vi "Analysis.Folders.Initialize.vi"(11 "Parameters in":T1) -> (3 "Parameters out":T1)   [LabVIEW 2015, in "NIAnalysis.lvlib"]
uses:
  NIAnalysis.lvlib
  Types/AnalysisGUI.Parameters.ctl
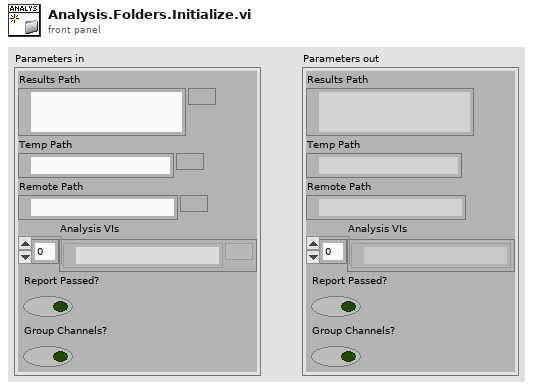
[diagram p1: front panel]
types:
  T1 = typedef "NIAnalysis.lvlib/AnalysisGUI.Parameters.ctl" = cluster{"Results Path":path, "Temp Path":path, "Remote Path":path, "Analysis VIs":path[], "Report Passed?":bool, "Group Channels?":bool}
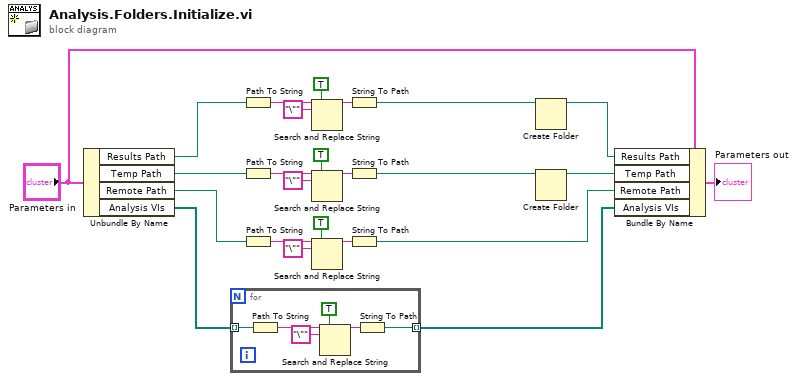
[diagram p0: block diagram]
diagram:
  n1 = Unbundle By Name("Parameters in") -> ("Results Path"=w2:path, "Temp Path"=w4:path, "Remote Path"=w6:path, "Analysis VIs"=w19:path[])
  n2 = for {
    tunnel: w19 -> [w26] mode=indexing
    tunnel: [w25] -> w23 mode=indexing
    n3 = Path To String(path=w26) -> (string=w29:string)
    n4 = Search and Replace String(replace all?=TRUE ("replace all? (F)"), input string=w29, search string="\"") -> (result string=w30:string)  [unwired: 5 in, 3 out]
    n5 = String To Path(string=w30) -> (path=w25:path)
  }
  n6 = Path To String(path=w2) -> (string=w17:string)
  n7 = Path To String(path=w4) -> (string=w13:string)
  n8 = Path To String(path=w6) -> (string=w9:string)
  n9 = Search and Replace String(replace all?=TRUE ("replace all? (F)"), input string=w17, search string="\"") -> (result string=w18:string)  [unwired: 5 in, 3 out]
  n10 = Search and Replace String(replace all?=TRUE ("replace all? (F)"), input string=w13, search string="\"") -> (result string=w14:string)  [unwired: 5 in, 3 out]
  n11 = Search and Replace String(replace all?=TRUE ("replace all? (F)"), input string=w9, search string="\"") -> (result string=w10:string)  [unwired: 5 in, 3 out]
  n12 = String To Path(string=w18) -> (path=w1:path)
  n13 = String To Path(string=w14) -> (path=w3:path)
  n14 = String To Path(string=w10) -> (path=w5:path)
  n15 = Create Folder(path (use dialog)=w1) -> (created path=w21:path)  [unwired: 2 in, 2 out]
  n16 = Create Folder(path (use dialog)=w3) -> (created path=w22:path)  [unwired: 2 in, 2 out]
  n17 = Bundle By Name(cluster="Parameters in", "Results Path"=w21, "Temp Path"=w22, "Remote Path"=w5, "Analysis VIs"=w23) -> (→"Parameters out":T1)
